vi "Read Address.vi"(8 "error in (no error)":errorcluster, 11 "ZI Lockin in":refnum<class "ZI Lockin.lvclass">) -> (0 "error out":errorcluster, 2 "Address":string, 3 "ZI Lockin out":refnum<class "ZI Lockin.lvclass">)   [LabVIEW 2016, in "ZI Lockin.lvclass"]
uses:
  ZI Lockin.lvclass
  ZI Lockin.lvclass/ZI Lockin.ctl
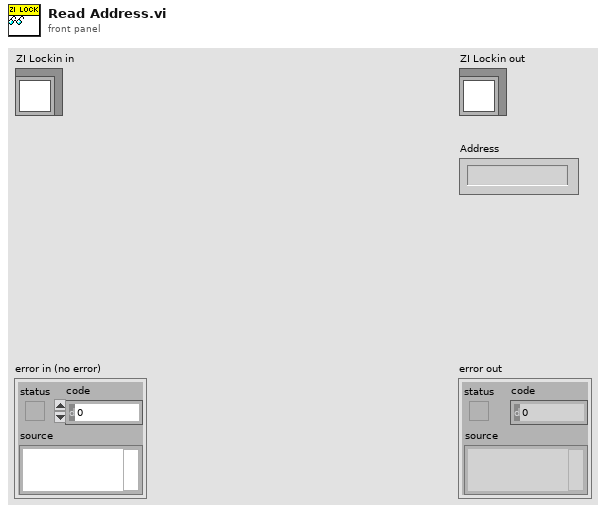
[diagram p1: front panel]
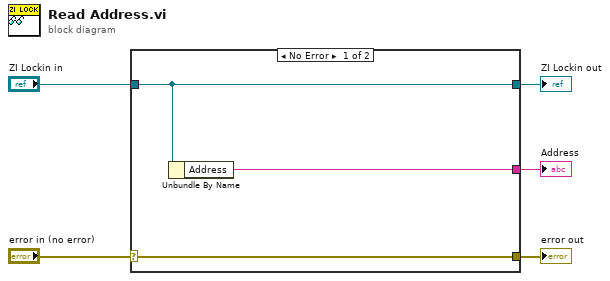
[diagram p0: block diagram]
diagram:
  n1 = case shown="No Error" "error in (no error)" {
    selector: "error in (no error)" -> [w8 w9]
    tunnel: [w8 w9] -> w4
    tunnel: [w7 w10] -> w2
    tunnel: "ZI Lockin in" -> [w7 w10]
    tunnel: [w6 _] -> w1
    frame No Error {
      n2 = Unbundle By Name(w7) -> ("Address"=w6:string)
    }
    frame Error {
    }
  }
  "error out" <- w4
  "ZI Lockin out" <- w2
  "Address" <- w1
